vi "sequential notify user.vi"(8 "error in":errorcluster, 11 "Msg":string) -> (0 "error out":errorcluster)   [LabVIEW 2020]
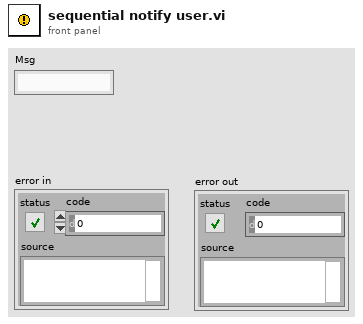
[diagram p1: front panel]
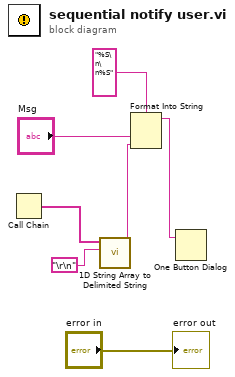
[diagram p0: block diagram]
diagram:
  n1 = Call Chain() -> (call chain=w6:string[])
  n2 = call <vilib>:"1D String Array to Delimited String.vi"("delimiter"="\r\n", "string array"=w6) -> ("delimited string"=w3:string)  [unwired: 9 in]
  n3 = Format Into String(format string="%S\n\n%S", "Msg", w3) -> (resulting string=w2:string)  [unwired: 2 in, 1 out]
  n4 = One Button Dialog(message=w2) -> ()  [unwired: 1 in, 1 out]
  "error out" <- "error in"
